vi "MaxDB.vi"(0 "dBCur":ext, 3 "db Prev":ext) -> (8 "Highest dB":ext)   [LabVIEW 2014]
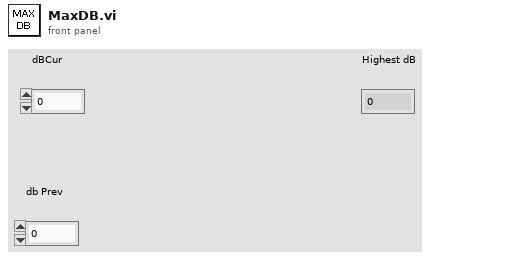
[diagram p1: front panel]
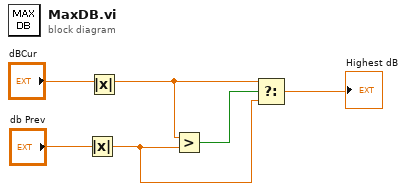
[diagram p0: block diagram]
diagram:
  n1 = Absolute Value(x="db Prev") -> (abs(x)=w1:ext)
  n2 = Absolute Value(x="dBCur") -> ()  [unwired: 1 out]
  n3 = Greater?(x="dBCur", y=w1) -> (0:w5:bool)
  n4 = Select(t="dBCur", s=w5, f=w1) -> (s? t:f=→"Highest dB":ext)
